vi "Read VIs.vi"(8 "error in (no error)":errorcluster, 11 "Library in":refnum<class "Library.lvclass">) -> (0 "error out":errorcluster, 2 "VIs":refnum<class "VI.lvclass">[](array[class]), 3 "Library out":refnum<class "Library.lvclass">)   [LabVIEW 2019, in "Library.lvclass"]
uses:
  Library.lvclass
  VI/VI.lvclass
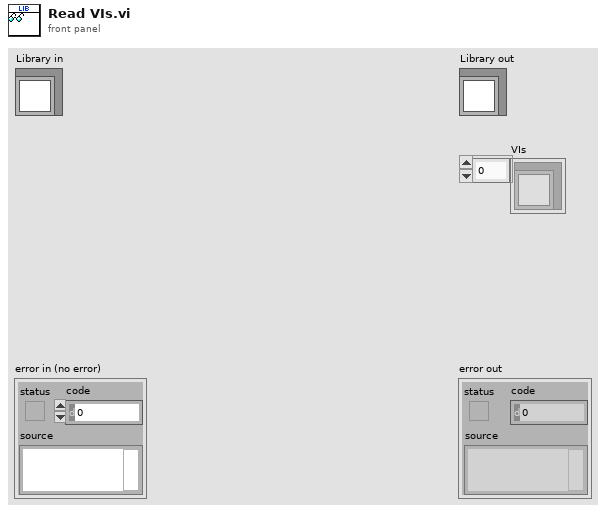
[diagram p1: front panel]
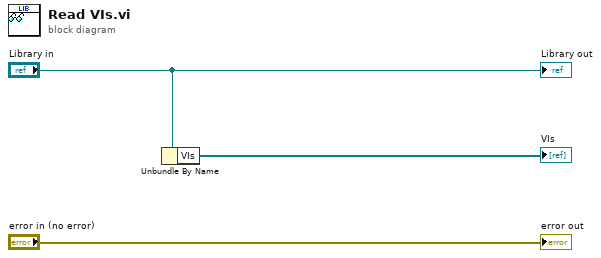
[diagram p0: block diagram]
diagram:
  n1 = Unbundle By Name("Library in") -> ("VIs"=→"VIs":refnum<class "VI.lvclass">[])
  "error out" <- "error in (no error)"
  "Library out" <- "Library in"
